vi "GUI Editor.vi"   [LabVIEW 2020]
panel:
  # "Loading GUI Editor..."
types:
  T1 = enum32{"Invalid", "Standard", "Closed", "Hidden", "Minimized", "Maximized"}
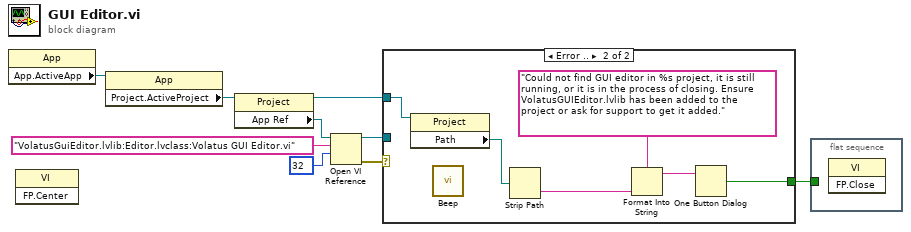
[diagram p0: block diagram]
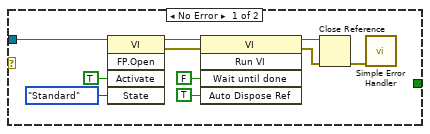
[diagram p2: hidden frame]
diagram:
  n1 = property class="App"() -> ("App.ActiveApp"=w5:refnum<vi>)  [unwired: 2 in, 2 out]
  n2 = invoke class="VI" method="FP.Center"() -> ()  [unwired: 3 in, 3 out]
  n3 = property class="App"(reference=w5) -> ("Project.ActiveProject"=w4:refnum<vi>)  [unwired: 1 in, 2 out]
  n4 = property class="Project"(reference=w4) -> (reference out=w2:refnum<vi>, "App Ref"=w3:refnum<vi>)  [unwired: 1 in, 1 out]
  n5 = Open VI Reference(application reference (local)=w3, vi path="VolatusGuiEditor.lvlib:Editor.lvclass:Volatus GUI Editor.vi", options=32) -> (vi reference=w6:refnum<vi>, error out=w7:errorcluster)  [unwired: 3 in]
  n6 = case shown="Error .." w7 {
    tunnel: w6 -> [w15 _]
    tunnel: w2 -> [_ w23]
    tunnel: [_ w20] -> w1
    frame No Error {
      n7 = invoke class="VI" method="FP.Open"(reference=w15, "Activate"=TRUE ("Activate?"), "State"=T1."Standard") -> (reference out=w12:refnum<vi>, error out=w11:errorcluster)  [unwired: 2 in, 3 out]
      n8 = invoke class="VI" method="Run VI"(reference=w12, error in=w11, "Wait until done"=FALSE ("Wait Until Done"), "Auto Dispose Ref"=TRUE ("Auto Dispose Reference")) -> (reference out=w17:refnum<vi>, error out=w16:errorcluster)  [unwired: 1 in, 3 out]
      n9 = Close Reference(reference=w17, error in (no error)=w16) -> (error out=w10:errorcluster)
      n10 = call <vilib>:"Simple Error Handler.vi"("error in (no error)"=w10) -> ()  [unwired: 4 in, 5 out]
    }
    frame Error {
      n11 = property class="Project"(reference=w23) -> ("Path"=w22:path)  [unwired: 1 in, 2 out]
      n12 = call <vilib>:"Beep.vi"() -> ()  [unwired: 12 in]
      n13 = Strip Path(path=w22) -> (name=w21:string)  [unwired: 1 out]
      n14 = Format Into String(format string="Could not find GUI editor in %s project, it is still running, or it is in the process of closing. Ensure VolatusGUIEditor.lvlib has been added to the project or ask for support to get it added.", w21) -> (resulting string=w24:string)  [unwired: 2 in, 1 out]
      n15 = One Button Dialog(message=w24) -> (true=w20:bool)  [unwired: 1 in]
    }
  }
  n16 = flat-sequence {
    tunnel: w1 -> [_]
    frame #0 {
      n17 = invoke class="VI" method="FP.Close"() -> ()  [unwired: 3 in, 3 out]
    }
  }
